vi "Interpolate pockels cell.vi"(8 "column":i32=1, 10 "nr of planes":i32=10 min=0 step=1, 11 "Data":dbl[][](array[numeric])=[[0.0, 1.0], [1.0, 2.700000047683716], [2.0, 7.400000095367432], [3.0, 150.0], [4.0, 80.0], [5.0, 220.0]] format="%0.2f") -> (2 "Interpolated Data":dbl[](array[numeric])=[0.0, 0.09090909090909091, 0.18181818181818182, 0.2727272727272727, 0.36363636363636365, 0.45454545454545453, 0.5454545454545454, 0.6363636363636364, 0.7272727272727273, 0.8181818181818182, 0.9090909090909091, 1.0, 1.0909090909090908, 1.1818181818181819, 1.2727272727272727, 1.3636363636363635, 1.4545454545454546, 1.5454545454545454, 1.6363636363636365, 1.7272727272727273, 1.8181818181818181, 1.9090909090909092, 2.0, 2.090909090909091, 2.1818181818181817, 2.272727272727273, 2.3636363636363638, 2.4545454545454546, 2.5454545454545454, 2.6363636363636362, 2.727272727272727, 2.8181818181818183, 2.909090909090909, 3.0, 3.090909090909091, 3.1818181818181817, 3.272727272727273, 3.3636363636363638, 3.4545454545454546, 3.5454545454545454, 3.6363636363636362, 3.727272727272727, 3.8181818181818183, 3.909090909090909, 4.0, 4.090909090909091, 4.181818181818182, 4.2727272727272725, 4.363636363636363, 4.454545454545454, 4.545454545454546, 4.636363636363637, 4.7272727272727275, 4.818181818181818, 4.909090909090909, 5.0] format="%0.2f", 3 "Raw Data and Interpolated Data":cluster{dbl[], "Best Exponential Fit":dbl[]}[](graph))   [LabVIEW 2012]
doc: "Determines the following types of interpolation: linear, polynomial, spline, and rational. You can enter the data on the front panel or read it from a file.\n\nNote: You must have the LabVIEW Full or Professional Development Systems to run this example."
uses:
  <vilib>/Analysis/NI_AALPro.lvlib
panel:
  # "x"
  # "y"
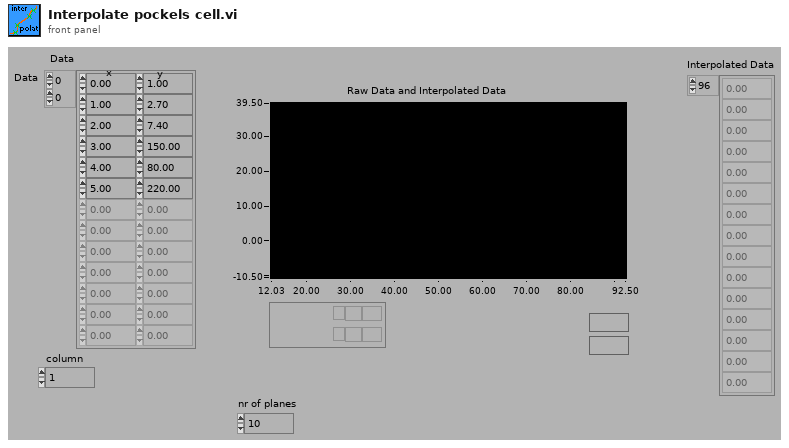
[diagram p1: front panel]
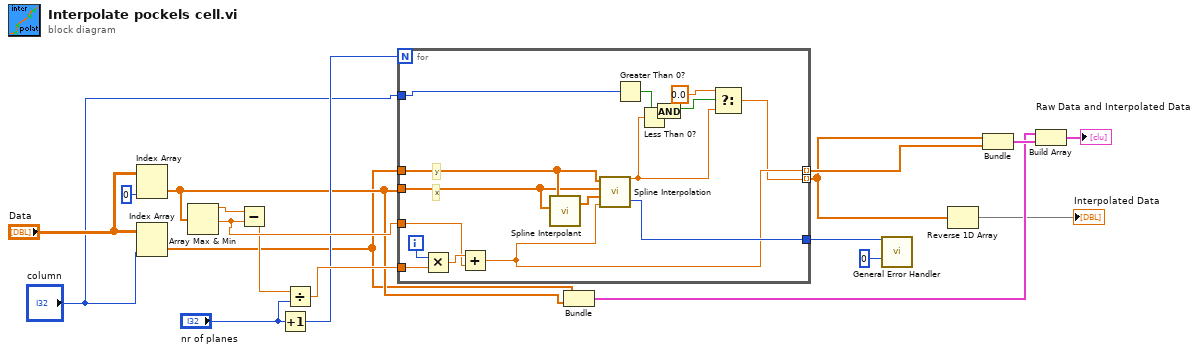
[diagram p0: block diagram]
diagram:
  n1 = Index Array(array="Data", index (col)=0) -> (element=w6:dbl[])  [unwired: 1 in]
  n2 = Index Array(array="Data", index (col)="column") -> (element=w5:dbl[])  [unwired: 1 in]
  n3 = Array Max & Min(array=w6) -> (max value=w9:dbl, min value=w10:dbl)  [unwired: 2 out]
  n4 = Subtract(x=w9, y=w10) -> (x-y=w7:dbl)
  n5 = Increment(x="nr of planes") -> (x+1=w8:i32)
  n6 = Divide(x=w7, y="nr of planes") -> (x/y=w12:dbl)
  n7 = for {
    N: w8 -> [_]
    tunnel: w5 -> [w35]
    tunnel: w6 -> [w31]
    tunnel: [w34] -> w19
    tunnel: w12 -> [w32]
    tunnel: [w23] -> w3 mode=indexing
    tunnel: [w28] -> w4 mode=indexing
    tunnel: w10 -> [w27]
    tunnel: "column" -> [w22]
    i -> [w33]
    # "x"
    # "y"
    n8 = Multiply(x=w33, y=w32) -> (x*y=w29:dbl)
    n9 = Add(x=w29, y=w27) -> (x+y=w28:dbl)
    n10 = call <vilib>:"Spline Interpolant.vi"("X"=w31, "Y"=w35) -> ("Interpolant"=w30:dbl[])  [unwired: 2 in, 1 out]
    n11 = call <vilib>:"Spline Interpolation.vi"("x value"=w28, "Interpolant"=w30, "X"=w31, "Y"=w35) -> ("error"=w34:i32, "interpolation value"=w24:dbl)
    n12 = Greater Than 0?(x=w22) -> (x > 0?=w20:bool)
    n13 = Less Than 0?(x=w24) -> (x < 0?=w25:bool)
    n14 = And(x=w20, y=w25) -> (x .and. y?=w21:bool)
    n15 = Select(t=0.0, s=w21, f=w24) -> (s? t:f=w23:dbl)
  }
  n16 = Bundle("Data"=w5, "Data"=w6) -> (w15:cluster{"Data":dbl[], "Data":dbl[]})  [unwired: 1 in]
  n17 = call <vilib>:"General Error Handler.vi"("[error code] (0)"=w19, "type of dialog (OK msg:1)"=0) -> ()  [unwired: 9 in, 5 out]
  n18 = Reverse 1D Array(array=w3) -> (reversed array=→"Interpolated Data":dbl[])
  n19 = Bundle(w3, w4) -> (w18:cluster{dbl[], dbl[]})  [unwired: 1 in]
  n20 = Build Array(w15, w18) -> (→"Raw Data and Interpolated Data":cluster{"Data":dbl[], "Data":dbl[]}[])
